vi "Pre-Init.vi"(8 "error in (no error)":errorcluster, 11 "Pulse Driver in":refnum<class "Pulse Driver.lvclass">) -> (0 "error out":errorcluster, 3 "Pulse Driver out":refnum<class "Pulse Driver.lvclass">)   [LabVIEW 2019, in "Pulse Driver.lvclass"]
uses:
  Pulse Driver.lvclass
  177aa3ad-ceef-4f55-896b-3dd49bc0a2ae.vi
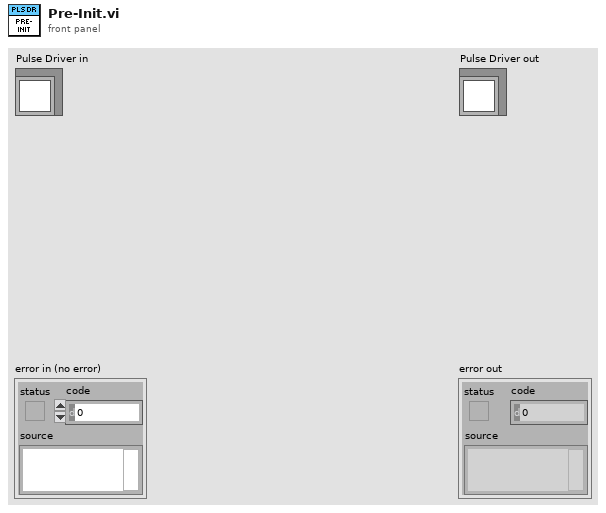
[diagram p1: front panel]
types:
  T1 = typedef "Pusle Driver Configuration.ctl" = cluster{"Pre-trigger duration":dbl, "Post-trigger duration":dbl, "Rate":dbl, "Ranges":dbl[], "Re-name channels":string[], "Active channels":string, "External clock":bool}
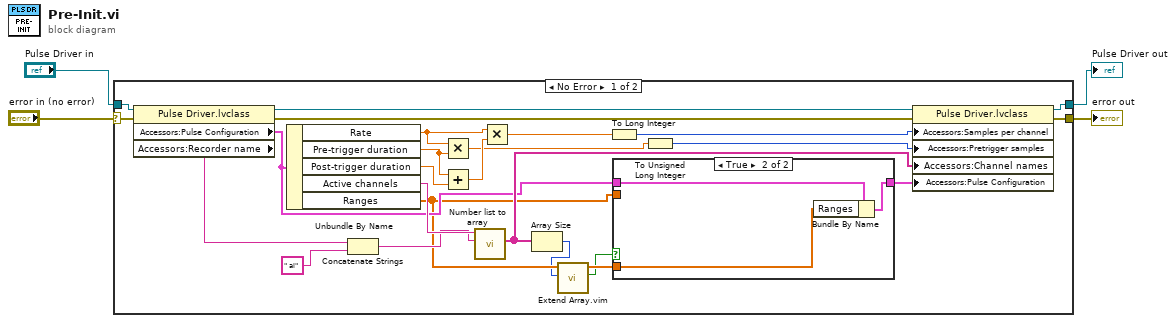
[diagram p0: block diagram]
diagram:
  n1 = case shown="No Error" "error in (no error)" {
    selector: "error in (no error)" -> [w17 w35]
    tunnel: [w16 w35] -> w3
    tunnel: [w26 w34] -> w1
    tunnel: "Pulse Driver in" -> [w29 w34]
    frame No Error {
      n2 = property class="Pulse Driver.lvclass"(reference=w29, error in=w17) -> (reference out=w28:refnum<class "Pulse Driver.lvclass">, error out=w18:errorcluster, "Accessors:Pulse Configuration"=w13:T1, "Accessors:Recorder name"=w11:string)
      n3 = Unbundle By Name(w13) -> ("Rate"=w19:dbl, "Pre-trigger duration"=w22:dbl, "Post-trigger duration"=w27:dbl, "Active channels"=w15:string, "Ranges"=w8:dbl[])
      n4 = Concatenate Strings(w11, " ai" ("Full names prefix")) -> (w9:string)
      n5 = Multiply(x=w19, y=w22) -> (x*y=w21:dbl)
      n6 = Add(x=w22, y=w27) -> (x+y=w24:dbl)
      n7 = call "Number list to array.vi"("Full names prefix"=w9, "Number list"=w15) -> ("Full names"=w14:string[])  [unwired: 8 in, 1 out]
      n8 = Multiply(x=w19, y=w24) -> (x*y=w23:dbl)
      n9 = Array Size(array=w14) -> (size(s)=w7:i32)
      n10 = call "Extend Array.vim"("Extend to size"=w7, "Array in"=w8) -> ("Extended"=w5:bool, "Array out"=w6:dbl[])  [unwired: 8 in]
      n11 = To Long Integer(number=w23) -> (32bit integer=w25:i32)
      n12 = case shown="True" w5 {
        tunnel: w8 -> [_ _]
        tunnel: w13 -> [w30 w33]
        tunnel: [w30 w32] -> w12
        tunnel: w6 -> [_ w31]
        frame False {
        }
        frame True {
          n13 = Bundle By Name(cluster=w33, "Ranges"=w31) -> (w32:T1)
        }
      }
      n14 = To Unsigned Long Integer(number=w21) -> (unsigned 32bit integer=w20:u32)
      n15 = property class="Pulse Driver.lvclass"(reference=w28, error in=w18, "Accessors:Samples per channel"=w25, "Accessors:Pretrigger samples"=w20, "Accessors:Channel names"=w14, "Accessors:Pulse Configuration"=w12) -> (reference out=w26:refnum<class "Pulse Driver.lvclass">, error out=w16:errorcluster)
    }
    frame Error {
    }
  }
  "error out" <- w3
  "Pulse Driver out" <- w1
